vi "Read Previous State.vi"(8 "error in (no error)":errorcluster, 11 "FW Arduino Control in":refnum<class "FW Arduino Control.lvclass">) -> (0 "error out":errorcluster, 2 "Previous State":i32[](array[numeric]), 3 "FW Arduino Control out":refnum<class "FW Arduino Control.lvclass">)   [LabVIEW 2024, in "FW Arduino Control.lvclass"]
uses:
  FW Arduino Control.lvclass
  Filter Wheel Object/Filter Wheel.lvclass
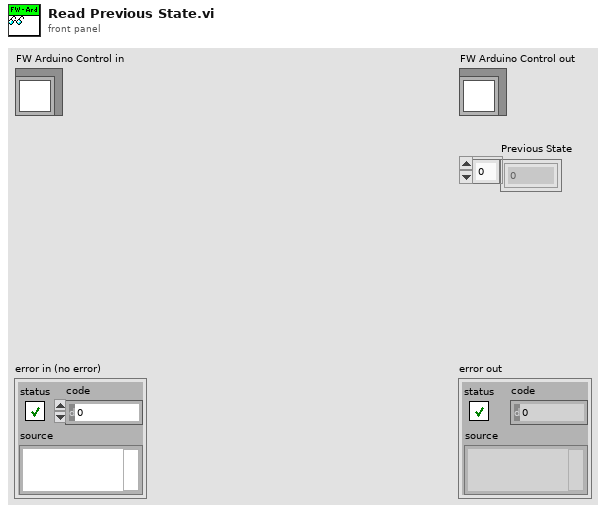
[diagram p1: front panel]
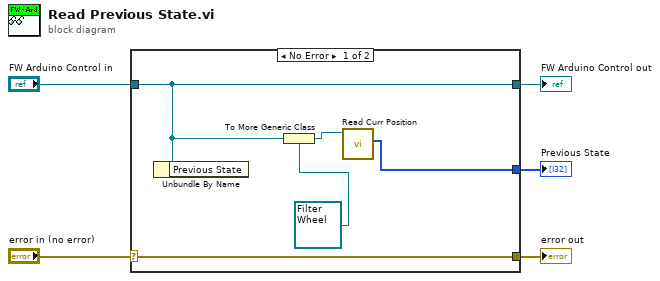
[diagram p0: block diagram]
diagram:
  n1 = case shown="No Error" "error in (no error)" {
    selector: "error in (no error)" -> [w10 w11]
    tunnel: [w10 w11] -> w4
    tunnel: [w9 w12] -> w2
    tunnel: "FW Arduino Control in" -> [w9 w12]
    tunnel: [w6 _] -> w1
    frame No Error {
      n2 = Unbundle By Name(w9) -> ()  [unwired: 1 out]
      n3 = To More Generic Class(target class=refnum<class "Filter Wheel.lvclass"> refnum ("Filter Wheel.lvclass"), reference=w9) -> (generic class reference=w7:refnum<class "Filter Wheel.lvclass">)
      n4 = call-dynamic "Read Curr Position.vi"("Filter Wheel in"=w7) -> ("Curr Position"=w6:i32[])  [unwired: 8 in, 2 out]
    }
    frame Error {
    }
  }
  "error out" <- w4
  "FW Arduino Control out" <- w2
  "Previous State" <- w1
